vi "Measurement.Uninit.vi"(8 "error in (no error)":errorcluster, 11 "Measurement.PhotocurrentMapping in":refnum<class "Measurement.PhotocurrentMapping.lvclass">) -> (0 "error out":errorcluster, 3 "Measurement.PhotocurrentMapping out":refnum<class "Measurement.PhotocurrentMapping.lvclass">)   [LabVIEW 2017, in "Measurement.PhotocurrentMapping.lvclass"]
uses:
  Measurement.PhotocurrentMapping.lvclass
  XYStage/XYStage.lvclass
  D:/upwork/Laser Measurement Tool/Laser/project/Subsystems/Device/Device.lvclass
  LIA/LIA.lvclass
  SMU/SMU.lvclass
  Device/Device.lvclass
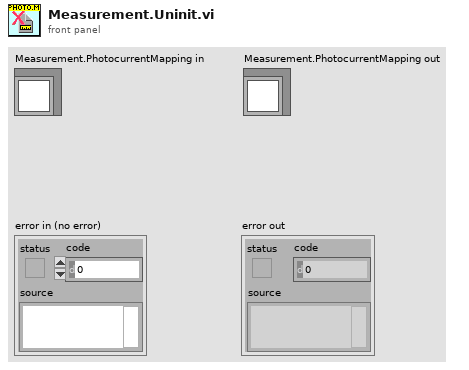
[diagram p1: front panel]
types:
  T1 = typedef "Measurement.PhotocurrentMapping.lvclass/Dependencies--Cluster.ctl" = cluster{"SMU":refnum<class "SMU.lvclass">, "LIA":refnum<class "LIA.lvclass">, "XYStage":refnum<class "XYStage.lvclass">}
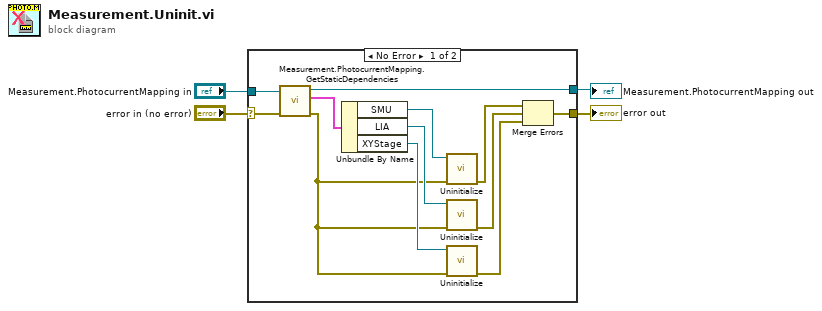
[diagram p0: block diagram]
diagram:
  n1 = case shown="No Error" "error in (no error)" {
    selector: "error in (no error)" -> [w15 w17]
    tunnel: "Measurement.PhotocurrentMapping in" -> [w16 w18]
    tunnel: [w14 w18] -> w2
    tunnel: [w5 w17] -> w1
    frame No Error {
      n2 = call "Measurement.PhotocurrentMapping.GetStaticDependencies.vi"("error in (no error)"=w15, "Measurement.PhotocurrentMapping in"=w16) -> ("error out"=w9:errorcluster, "Dependencies"=w13:T1, "Measurement.PhotocurrentMapping out"=w14:refnum<class "Measurement.PhotocurrentMapping.lvclass">)  [unwired: 7 in]
      n3 = Unbundle By Name(w13) -> ("SMU"=w12:refnum<class "SMU.lvclass">, "LIA"=w11:refnum<class "LIA.lvclass">, "XYStage"=w10:refnum<class "XYStage.lvclass">)
      n4 = call "Uninitialize.vi"("error in (no error)"=w9, "Device in"=w12) -> ("error out"=w8:errorcluster)  [unwired: 8 in, 1 out]
      n5 = call "Uninitialize.vi"("error in (no error)"=w9, "Device in"=w11) -> ("error out"=w7:errorcluster)  [unwired: 8 in, 1 out]
      n6 = call "Uninitialize.vi"("error in (no error)"=w9, "Device in"=w10) -> ("error out"=w6:errorcluster)  [unwired: 8 in, 1 out]
      n7 = Merge Errors(w8, w7, w6) -> (w5:errorcluster)
    }
    frame Error {
    }
  }
  "error out" <- w1
  "Measurement.PhotocurrentMapping out" <- w2
